vi "SetCellColor__slk_tc.vi"(0 "tree control in":refnum<class "TreeControl.lvclass">, 5 "input tag (current tag)":string, 9 "cell color (white)":u32(colorbox)=16777215, 11 "error in (no error)":errorcluster, 12 "column # (entire row=-2)":i32=-2) -> (4 "tree control out":refnum<class "TreeControl.lvclass">, 6 "output tag":string, 15 "error out":errorcluster)   [LabVIEW 2020, in "TreeControl.lvclass"]
doc: "Sets cell color of input tag with specified column."
uses:
  Library/TreeControl.lvclass
  Library/TreeControl.lvclass/TreeControl.ctl
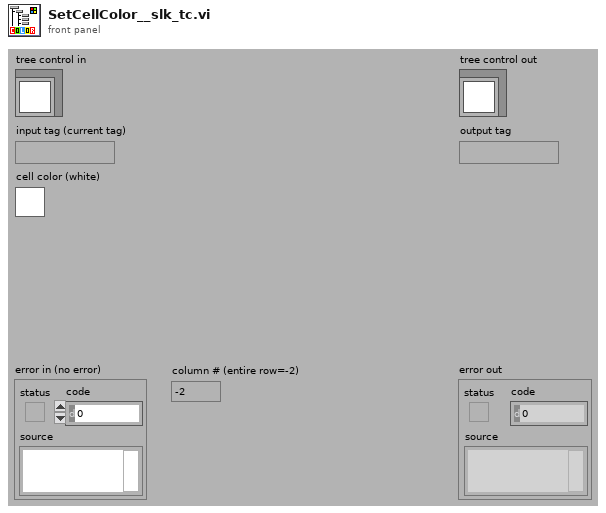
[diagram p1: front panel]
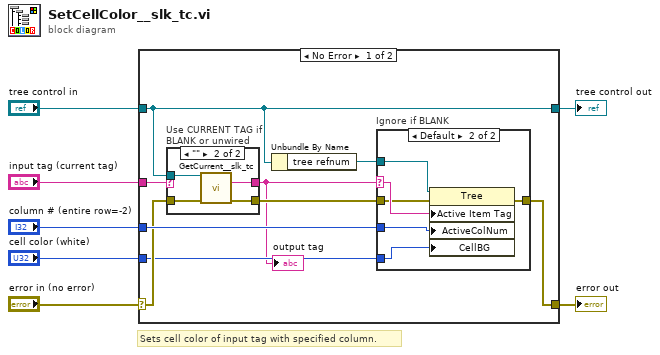
[diagram p0: block diagram]
diagram:
  # "Sets cell color of input tag with specified column."
  n1 = case shown="No Error" "error in (no error)" {
    selector: "error in (no error)" -> [w11 w31]
    tunnel: [w10 w31] -> w6
    tunnel: [w15 w30] -> w4
    tunnel: "tree control in" -> [w15 w30]
    tunnel: "input tag (current tag)" -> [w16 _]
    tunnel: "column # (entire row=-2)" -> [w13 _]
    tunnel: "cell color (white)" -> [w9 _]
    frame No Error {
      n2 = case "Use CURRENT TAG if BLANK or unwired" shown="\"\"" w16 {
        selector: w16 -> [w25 _]
        tunnel: [w25 w29] -> w8
        tunnel: w15 -> [_ w28]
        tunnel: w11 -> [w24 w27]
        tunnel: [w24 w26] -> w12
        frame Default {
        }
        frame "" {
          n3 = call "GetCurrent__slk_tc.vi"("tree control in"=w28, "error in (no error)"=w27) -> ("current tag"=w29:string, "error out"=w26:errorcluster)  [unwired: 1 in, 11 out]
        }
      }
      "output tag" <- w8
      n4 = Unbundle By Name(w15) -> ("tree refnum"=w14:refnum<vi>)
      n5 = case "Ignore if BLANK" shown="Default" w8 {
        selector: w8 -> [_ w22]
        tunnel: w14 -> [_ w23]
        tunnel: w13 -> [_ w21]
        tunnel: w12 -> [w17 w20]
        tunnel: [w17 w19] -> w10
        tunnel: w9 -> [_ w18]
        frame "" {
        }
        frame Default {
          n6 = property class="Tree"(reference=w23, error in=w20, "Active Item Tag"=w22, "ActiveColNum"=w21, "CellBG"=w18) -> (error out=w19:errorcluster)  [unwired: 1 out]
        }
      }
    }
    frame Error {
    }
  }
  "error out" <- w6
  "tree control out" <- w4
